vi "Create Accessor VIs.vi"   [LabVIEW 2011, in "Generator.lvlib"]
uses:
  C:/Program Files (x86)/National Instruments/LabVIEW 2011/resource/Framework/Providers/LVClassLibrary/NewAccessors/BaseAccessorScripter/BaseAccessorScripter.lvclass
  Generator.lvlib
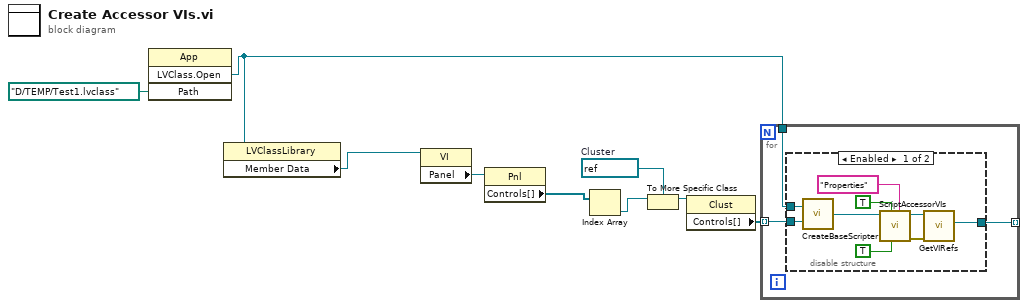
[diagram p0: block diagram]
diagram:
  w4 = refnum<vi> refnum  # Cluster
  n1 = invoke class="App" method="LVClass.Open"("Path"=path "D:/TEMP/Test1.lvclass") -> ("LVClass.Open"=w1:refnum<vi>)  [unwired: 3 in, 3 out]
  n2 = property class="LVClassLibrary"(reference=w1) -> ("Member Data"=w8:refnum<vi>)  [unwired: 1 in, 2 out]
  n3 = property class="VI"(reference=w8) -> ("Panel"=w7:refnum<vi>)  [unwired: 1 in, 2 out]
  n4 = property class="Pnl"(reference=w7) -> ("Controls[]"=w6:refnum<vi>[])  [unwired: 1 in, 2 out]
  n5 = Index Array(array=w6) -> (element=w5:refnum<vi>)  [unwired: 1 in]
  n6 = To More Specific Class(target class=w4, reference=w5) -> (specific class reference=w3:refnum<vi>)  [unwired: 1 in, 1 out]
  n7 = property class="Clust"(reference=w3) -> ("Controls[]"=w2:refnum<vi>[])  [unwired: 1 in, 2 out]
  n8 = for {
    tunnel: w2 -> [w12] mode=indexing
    tunnel: w1 -> [w11]
    tunnel: [w10] -> _ mode=indexing
    n9 = disable-structure shown="Enabled" {
      disable-tunnel: w11 -> [w17 _]
      disable-tunnel: w12 -> [w16 _]
      disable-tunnel: [w13 _] -> w10
      frame Enabled {
        n10 = call "CreateBaseScripter.vi"("Ctl Refnum"=w16, "LVClassLibrary Ref"=w17) -> ("Scripter Out"=w21:refnum<class "BaseAccessorScripter.lvclass">)
        n11 = call-dynamic "ScriptAccessorVIs.vi"("Virtual Folder Name"="Properties", "Create as Properties"=TRUE, "Include error terminals"=TRUE, "BaseAccessorScripter in"=w21) -> ("error out"=w14:errorcluster, "BaseAccessorScripter out"=w15:refnum<class "BaseAccessorScripter.lvclass">)  [unwired: 6 in]
        n12 = call-dynamic "GetVIRefs.vi"("error in (no error)"=w14, "BaseAccessorScripter in"=w15) -> ("Read VI"=w13:refnum<vi>)  [unwired: 6 in, 3 out]
      }
      frame Disabled {
      }
    }
  }
